vi "Read Lift Encoders.vi"(1 "Input Array":dbl[](array[numeric])) -> (0 "Appended Array":dbl[](array[numeric]))   [LabVIEW 2014]
uses:
  Begin/Global RefNums.vi
panel:
  out "Lift Right Rate [counts/sec]":dbl
  out "Lift Right Height [counts]":dbl
  out "Lift Left Rate [counts/sec]":dbl
  out "Lift Left Height [counts]":dbl
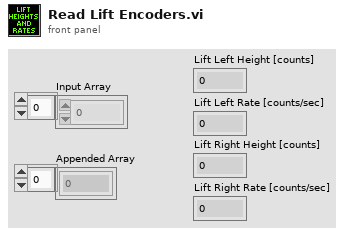
[diagram p1: front panel]
types:
  T1 = typedef "WPI_EncoderDevRef.ctl" = cluster{"DevStatus":errorcluster, "EncoderIndex":T2, "CounterIndex":T3, "DistancePerCount":dbl, "Decoding Type":T4}
  T2 = typedef "FPGA_EncoderIdx.ctl" = enum8{"Enc 0", "Enc 1", "Enc 2", "Enc 3", "Enc 4", "Enc 5", "Enc 6", "Enc 7", "Invalid"}
  T3 = typedef "FPGA_CounterCtrSystemIndex.ctl" = enum8{"Ctr 0", "Ctr 1", "Ctr 2", "Ctr 3", "Ctr 4", "Ctr 5", "Ctr 6", "Ctr 7", "Invalid"}
  T4 = typedef "WPI_EncoderType.ctl" = enum16{"1x", "2x", "4x"}
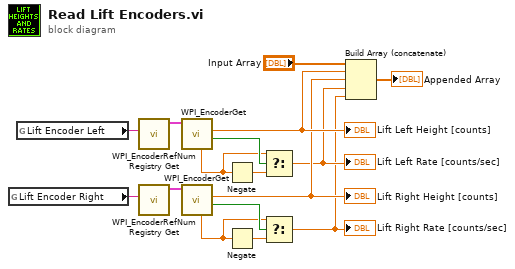
[diagram p0: block diagram]
diagram:
  n1 = global read "Global RefNums.vi" "Lift Encoder Right"() -> (w14:string)
  n2 = global read "Global RefNums.vi" "Lift Encoder Left"() -> (w15:string)
  n3 = call <vilib>:"WPI_EncoderRefNum Registry Get.vi"("refnum name"=w15) -> ("EncoderDevRef"=w16:T1)  [unwired: 9 in, 1 out]
  n4 = call <vilib>:"WPI_EncoderRefNum Registry Get.vi"("refnum name"=w14) -> ("EncoderDevRef"=w13:T1)  [unwired: 9 in, 1 out]
  n5 = call <vilib>:"WPI_EncoderGet.vi"("EncoderDevRef"=w16) -> ("Direction"=w11:bool, "Distance"=w4:dbl, "Rate"=w7:dbl)  [unwired: 5 in, 3 out]
  "Lift Left Height [counts]" <- w4
  n6 = call <vilib>:"WPI_EncoderGet.vi"("EncoderDevRef"=w13) -> ("Direction"=w12:bool, "Distance"=w3:dbl, "Rate"=w8:dbl)  [unwired: 5 in, 3 out]
  "Lift Right Height [counts]" <- w3
  n7 = Negate(x=w7) -> (-x=w9:dbl)
  n8 = Negate(x=w8) -> (-x=w10:dbl)
  n9 = Select(t=w7, s=w11, f=w9) -> (s? t:f=w2:dbl)
  "Lift Left Rate [counts/sec]" <- w2
  n10 = Select(t=w8, s=w12, f=w10) -> (s? t:f=w1:dbl)
  "Lift Right Rate [counts/sec]" <- w1
  n11 = Build Array (concatenate)("Input Array", w4, w3, w2, w1) -> (→"Appended Array":dbl[])
